vi "MD420_ACT_SetpointFormation.vi"() -> ()   [LabVIEW 2022 SP3, in "MD420.lvclass"]
uses:
  MD420.lvclass
  MD420.lvclass/MD420.ctl
panel:
  in  "Target value":dbl
  in  "Matching":bool
  in  "-0.9 K/min":bool
  in  "Rels +0.6 K/min":bool
  in  "TVal reached":bool
  in  "Target Grad":dbl
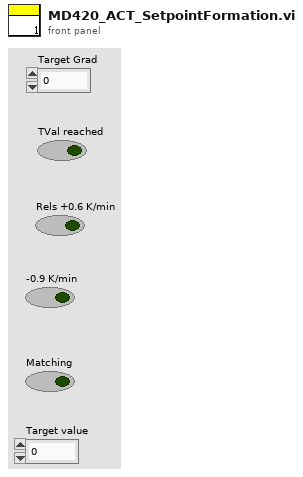
[diagram p1: front panel]
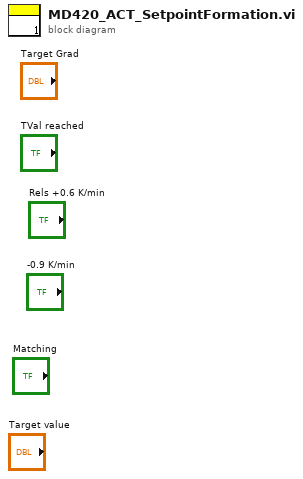
[diagram p0: block diagram]
diagram:
